vi "Read Data as Mono12p Image.vi"(8 "error in (no error)":errorcluster, 11 "Buffer in":refnum<class "Buffer.lvclass">) -> (0 "error out":errorcluster, 2 "Image":u16[][](array[numeric]), 3 "Buffer":refnum<class "Buffer.lvclass">)   [LabVIEW 2020, in "Buffer.lvclass"]
doc: "Read the buffer data assuming it is in the Mono 12 Packed pixel format and return it as a 2D array of U16s."
uses:
  Buffer.lvclass
  Buffer.lvclass/Buffer.ctl
  bin/gindustrialcam_32-1.dll
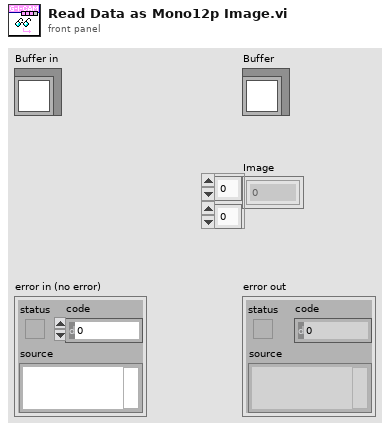
[diagram p1: front panel]
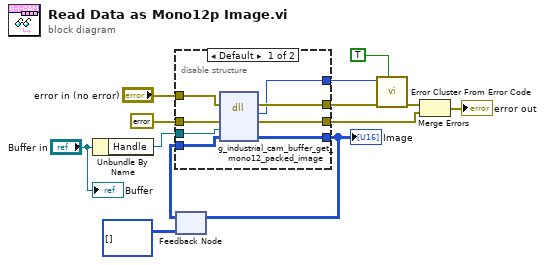
[diagram p0: block diagram]
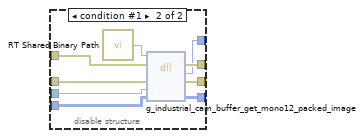
[diagram p2: hidden frame]
diagram:
  n1 = Unbundle By Name("Buffer in") -> ("Handle"=w10:refnum<data-value>)
  n2 = feedback #1(u16[][] [] ("Image")) -> (w8:u16[][])
  n3 = disable-structure shown="Default" {
    disable-tunnel: "error in (no error)" -> [w21 w30]
    disable-tunnel: w10 -> [w20 w29]
    disable-tunnel: w8 -> [w19 w28]
    disable-tunnel: [w18 w27] -> w7
    disable-tunnel: [w17 w26] -> w6
    disable-tunnel: [w16 w25] -> w4
    disable-tunnel: errorcluster {"status"=FALSE, "code"=0, "source"=""} ("error constant") -> [w15 w24]
    disable-tunnel: [w14 w23] -> w1
    frame condition #0 (active) {
      n4 = dll-call lib="C:/serenial/lib/g-industrial-camera/LabVIEW/g_industrial_cam/bin/gindustrialcam_*-1.*" fn="g_industrial_cam_buffer_get_mono12_packed_image"(error in=w21, "err"=w15, "edvr"=w20, "image"=w19) -> (error out=w18:errorcluster, "Mg_Error"=w17:i32, "err"=w16:errorcluster, "image"=w14:u16[][])  [unwired: 3 in, 1 out]
    }
    frame condition #1 {
      n5 = call "RT Shared Binary Path.vi"() -> ("Path"=w22:path)
      n6 = dll-call lib="C:/serenial/lib/g-industrial-camera/LabVIEW/g_industrial_cam/bin/gindustrialcam_*-1.*" fn="g_industrial_cam_buffer_get_mono12_packed_image"(path in=w22, error in=w30, "err"=w24, "edvr"=w29, "image"=w28) -> (error out=w27:errorcluster, "Mg_Error"=w26:i32, "err"=w25:errorcluster, "image"=w23:u16[][])  [unwired: 2 in, 1 out]
    }
  }
  "Image" <- w1
  n7 = feedback-in #1(w1) -> ()
  n8 = call <vilib>:"Error Cluster From Error Code.vi"("show call chain? (False)"=TRUE, "error in (no error)"=w7, "error code (0)"=w6) -> ("error out"=w5:errorcluster)  [unwired: 6 in]
  n9 = Merge Errors(w5, w4) -> (→"error out":errorcluster)
  "Buffer" <- "Buffer in"
